vi "AB_API Do Two Step Build.vi"(8 "error in (no error)":errorcluster, 11 "Build in":refnum<class "AB_Build.lvclass">) -> (0 "error out":errorcluster, 1 "Dependencies":T1[](array[typedef]), 2 "GeneratedFiles":path[](array[path]), 3 "Build out":refnum<class "AB_Build.lvclass">)   [LabVIEW 2020]
uses:
  <vilib>/AppBuilder/AB_Classes/Build/AB_Build.lvclass
  <vilib>/AppBuilder/AB_Dependency.ctl
  <vilib>/Utility/lvfile.llb/LVFileType.ctl
  <vilib>/Utility/lvfile.llb/NI_FileType.lvlib
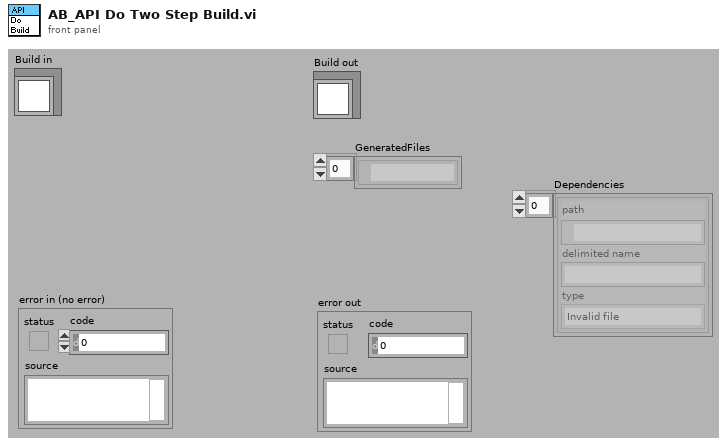
[diagram p1: front panel]
types:
  T1 = typedef "AB_Dependency.ctl" = cluster{"path":path, "delimited name":string, "type":T2}
  T2 = typedef "NI_FileType.lvlib/LVFileType.ctl" = enum32{"Invalid file", "Unknown type", "Instrument", "Control", "Polymorphic VI", "Project", "Library", "LVClass", "XControl", "XNode", "Shared library", ".NET assembly", "ActiveX interface", "CIN", "Run-time menu", "Palette menu", "Help file", "LLB", "XNode Edit Dependency", "Class Private Data Control", "Statechart", "MathScript .m file", "Ladder Diagram", "LVLibp", "XNode Build Dependency"}
  T3 = typedef "AB_Build.ctl" = cluster{"buildSpecName":string, "buildSpecDescription":string, "destinations":refnum<class "AB_Destination.lvclass">[], "exclusionOption":T4, "defaultLanguage":string, "supportedLanguages":string[], "excludedDirectories":path[], "buildContext":refnum<vi>, "buildObject":T5, "preview":bool, "programatic":bool, "progressBarEvents":T6, "userLog_Path":path, "preActionID":string, "preAction_Path":path, "postActionID":string, "postAction_Path":path, "eng_checkForBrokenVIs?":bool, "eng_verboseLinkerErrors?":bool, "localDest_Path":path, "targetDest_Path":path, "removeVIObject":u16, "cache":refnum<class "PreviewCache.lvclass">, "use cache":bool, "previewCache_ID":string, "buildCache_ID":string, "eng_TempLocalDest_Path":path, "eng_collectDependencies?":bool, "versionInfo":cluster{"buildVersion":cluster{"major":u16, "minor":u16, "patch":u16, "build":u16}, "autoIncrement":bool}, "eng_enableVIChecksums":bool}
  T4 = typedef "AB_Exclusion_Option.ctl" = cluster{"typedefs":bool, "polymorphicVIs":bool, "unusedLibraryItems":bool, "modifyLibraryFile":bool, "edit-timeDependencies":bool, "inlineVIs":bool, "dependent PPLs":bool, "dependent DLLs":bool}
  T5 = typedef "ItemRef.ctl" = u64
  T6 = typedef "provcom_ProgressBar_Events.ctl" = cluster{"newJob":refnum<user-event>, "newItem":refnum<user-event>, "errorMsg":T7, "cancel":refnum<user-event>}
  T7 = typedef "mxLvBuildError.ctl" = refnum<user-event>
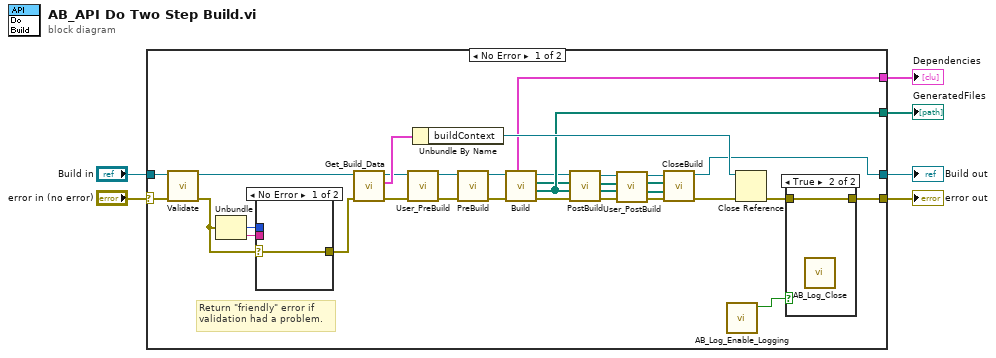
[diagram p0: block diagram]
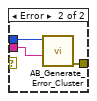
[diagram p2: hidden frame]
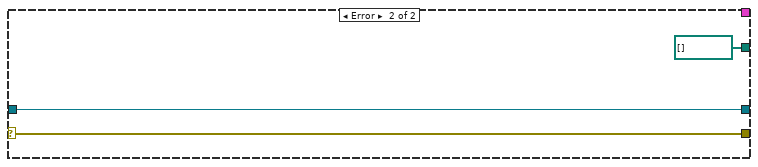
[diagram p4: hidden frame]
diagram:
  n1 = case shown="No Error" "error in (no error)" {
    selector: "error in (no error)" -> [w11 w48]
    tunnel: "Build in" -> [w10 w47]
    tunnel: [w23 path[] [] ("GeneratedFiles")] -> w5
    tunnel: [w18 w48] -> w4
    tunnel: [w16 w47] -> w3
    tunnel: [w7 _] -> w1
    frame No Error {
      # "Return \"friendly\" error if \nvalidation had a problem."
      n2 = call-dynamic "Validate.vi"("error in (no error)"=w11, "Build in"=w10) -> ("error out"=w14:errorcluster, "Build out"=w9:refnum<class "AB_Build.lvclass">)  [unwired: 8 out]
      n3 = Unbundle(w14) -> ("code"=w12:i32, "source"=w13:string)  [unwired: 1 out]
      n4 = case shown="No Error" w14 {
        selector: w14 -> [w40 _]
        tunnel: w12 -> [_ w43]
        tunnel: w13 -> [_ w42]
        tunnel: [w40 w41] -> w8
        frame No Error {
        }
        frame Error {
          n5 = call <vilib>:"AB_Generate_Error_Cluster.vi"("Additional Message"=w42, "Code"=w43) -> ("error out"=w41:errorcluster)  [unwired: 2 in, 7 out]
        }
      }
      n6 = call <vilib>:"Get_Build_Data.vi"("error in (no error)"=w8, "Class in"=w9) -> ("error out"=w37:errorcluster, "data"=w38:T3, "Class out"=w36:refnum<class "AB_Build.lvclass">)  [unwired: 7 out]
      n7 = call-dynamic "User_PreBuild.vi"("error in (no error)"=w37, "Build in"=w36) -> ("error out"=w26:errorcluster, "Build out"=w25:refnum<class "AB_Build.lvclass">)  [unwired: 8 in]
      n8 = Unbundle By Name(w38) -> ("buildContext"=w39:refnum<vi>)
      n9 = call-dynamic "PreBuild.vi"("error in (no error)"=w26, "Build in"=w25) -> ("error out"=w20:errorcluster, "Build out"=w19:refnum<class "AB_Build.lvclass">)  [unwired: 1 in, 7 out]
      n10 = call-dynamic "Build.vi"("error in (no error)"=w20, "Build in"=w19) -> ("error out"=w24:errorcluster, "GeneratedFiles"=w23:path[], "GeneratedDirectories"=w22:path[], "Build out"=w21:refnum<class "AB_Build.lvclass">, "Dependencies"=w7:T1[])  [unwired: 5 out]
      n11 = call-dynamic "PostBuild.vi"("error in (no error)"=w24, "GeneratedFiles in"=w23, "GeneratedDirectories in"=w22, "Build in"=w21) -> ("error out"=w27:errorcluster, "GeneratedFiles out"=w34:path[], "GeneratedDirectories out"=w33:path[], "Build out"=w28:refnum<class "AB_Build.lvclass">)  [unwired: 4 out]
      n12 = call-dynamic "User_PostBuild.vi"("error in (no error)"=w27, "GeneratedFiles in"=w34, "GeneratedDirectories in"=w33, "Build in"=w28) -> ("error out"=w30:errorcluster, "GeneratedFiles out"=w31:path[], "GeneratedDirectories out"=w32:path[], "Build out"=w29:refnum<class "AB_Build.lvclass">)  [unwired: 4 in]
      n13 = call-dynamic "CloseBuild.vi"("error in (no error)"=w30, "GeneratedFiles"=w31, "GeneratedDirectories"=w32, "Build in"=w29) -> ("error out"=w15:errorcluster, "Build out"=w16:refnum<class "AB_Build.lvclass">)  [unwired: 6 out]
      n14 = call <vilib>:"AB_Log_Enable_Logging.vi"() -> ("log?"=w35:bool)  [unwired: 2 in, 9 out]
      n15 = Close Reference(reference=w39, error in (no error)=w15) -> (error out=w17:errorcluster)
      n16 = case shown="True" w35 {
        tunnel: [w44 w45] -> w18
        tunnel: w17 -> [w44 w45]
        frame False {
        }
        frame True {
          n17 = call <vilib>:"AB_Log_Close.vi"() -> ()  [unwired: 1 in, 11 out]
        }
      }
    }
    frame Error {
    }
  }
  "GeneratedFiles" <- w5
  "error out" <- w4
  "Build out" <- w3
  "Dependencies" <- w1
